vi "transform_points.vi"(8 "Transform":T1, 10 "Points":sgl[][](array[numeric])) -> (2 "Transformed points":sgl[][](array[numeric]))   [LabVIEW 2013]
uses:
  <vilib>/Analysis/Matrix/Datatypes/RealMatrix.ctl
  <vilib>/Analysis/baseanly.llb/A x Vector.vi
  <vilib>/Analysis/NI_AALBase.lvlib
  <vilib>/Analysis/Matrix/NI_Matrix.lvlib
panel:
  # "Given  Nx3 array of points, transform by a 4x4 linear homogenous transform.  The points are implicitly padded with a 1 so that they are translated as well as rotated."
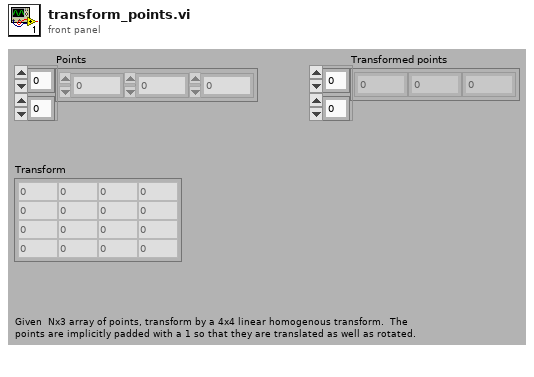
[diagram p1: front panel]
types:
  T1 = typedef "NI_Matrix.lvlib/RealMatrix.ctl" = dbl[][]
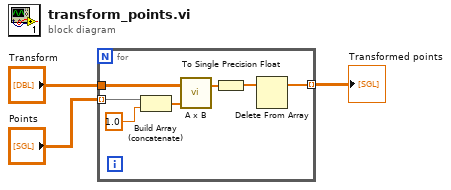
[diagram p0: block diagram]
diagram:
  n1 = for {
    tunnel: "Points" -> [w6] mode=indexing
    tunnel: "Transform" -> [w5]
    tunnel: [w4] -> w1 mode=indexing
    n2 = Build Array (concatenate)(w6, sgl 1.0) -> (w9:sgl[])
    n3 = call-poly <vilib>:"A x B.vi"("Vector"=w9, "A"=w5) -> ("A x Vector"=w7:dbl[])  [unwired: 1 out]
    n4 = To Single Precision Float(number=w7) -> (single precision float=w10:sgl[])
    n5 = Delete From Array(array=w10) -> (array with subset deleted=w4:sgl[])  [unwired: 2 in, 1 out]
  }
  "Transformed points" <- w1
